vi "Read.vi"(8 "error in (no error)":errorcluster, 11 "Double Float.lvclass in":refnum<class "Reciprocal_Numeric.lvclass">) -> (0 "error out":errorcluster, 2 "Value":T1, 3 "Double Float.lvclass out":refnum<class "Reciprocal_Numeric.lvclass">)   [LabVIEW 2021, in "Reciprocal_Numeric.lvclass"]
uses:
  Reciprocal_Numeric.lvclass
  Abs_Types/Double Float/Support/Type.ctl
  Reciprocal_Numeric.lvclass/Reciprocal_Numeric.ctl
  Abs_Types/Numeric/Abs_Numeric.lvclass
  Abs_Types/Double Float/Abs_Double Float.lvclass
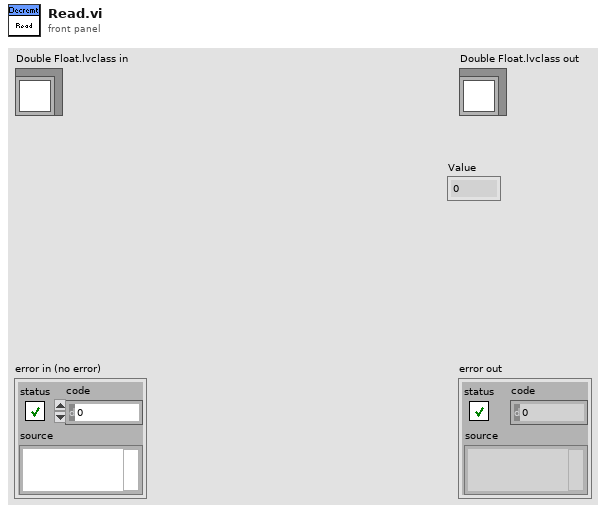
[diagram p1: front panel]
types:
  T1 = typedef "Abs_Double Float.lvclass/Type.ctl" = dbl
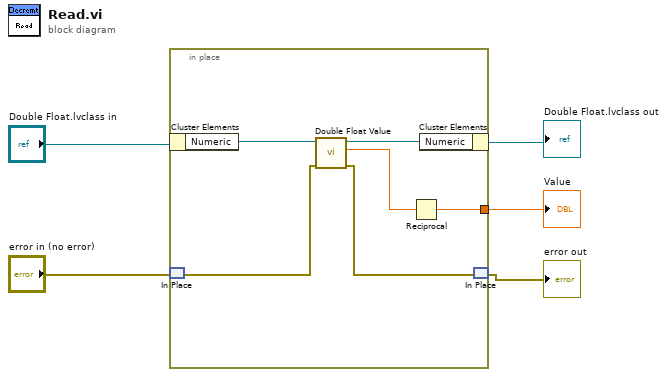
[diagram p0: block diagram]
diagram:
  n1 = in-place {
    in-place-border: [w8] -> w4
    n2 = in-place-cluster #1("Double Float.lvclass in") -> ("Numeric"=w11:refnum<class "Abs_Numeric.lvclass">)
    n3 = in-place-match #2("error in (no error)") -> (w7:errorcluster)
    n4 = call-dynamic "Double Float Value.vi"("error in (no error)"=w7, "Numeric in"=w11) -> ("error out"=w6:errorcluster, "Double"=w9:dbl, "Numeric out"=w10:refnum<class "Abs_Numeric.lvclass">)  [unwired: 7 in]
    n5 = Reciprocal(x=w9) -> (1/x=w8:dbl)
    n6 = in-place-cluster #1("Numeric"=w10) -> (→"Double Float.lvclass out":refnum<class "Reciprocal_Numeric.lvclass">)
    n7 = in-place-match #2(w6) -> (→"error out":errorcluster)
  }
  "Value" <- w4
